vi "LS336_config.vi"(0 "VISA Refnum in":refnum<visa-resource-name>, 1 "Enable Setpoint (F:Off)":bool, 2 "Mode (0:Off)":u16(ring) items=["Off", "Closed Loop PID", "Zone", "Open Loop"], 3 "Rate (D) (0.0 %)":dbl format="%.1f", 4 "Input (0:None)":u16(ring) items=["None", "A", "B", "C", "D"], 5 "Heater Resistance (1:25 Ohms)":u16(ring)=1 items=["25 Ohms"=1, "50 Ohms"=2], 6 "Max Current (0:User Specified)":u16(ring) items=["User Specified", "0.707 A", "1.0 A", "1.141 A", "2.0 A"], 8 "Output's Control Loop (1:1)":u16(ring)=1 items=["1"=1, "2"=2], 9 "Gain (P) (50.0)":dbl=50.0 format="%.1f", 10 "Power Up Enable (F: Off)":bool, 11 "Heater Out Display (1:Current)":u16(ring)=1 items=["Current"=1, "Power"=2], 12 "Manual Output (0.00 %)":dbl format="%.2f", 13 "Max User Current (2.000)":dbl=2.0 format="%.3f", 14 "Range (0:Off)":u16(ring) items=["Off", "Low (On)", "Medium", "High"], 15 "Reset (I) (20.0)":dbl=20.0 format="%.1f", 16 "Setpoint (0.00000)":dbl format="%.5f") -> ()   [LabVIEW 2017]
uses:
  <instrlib>/Lake Shore 336/Lake Shore 336.lvlib
panel:
  in  "Setpoint Ramping \nEnable (F: Off)":bool
  in  "Ramp Rate (0.0)":dbl format="%.1f"
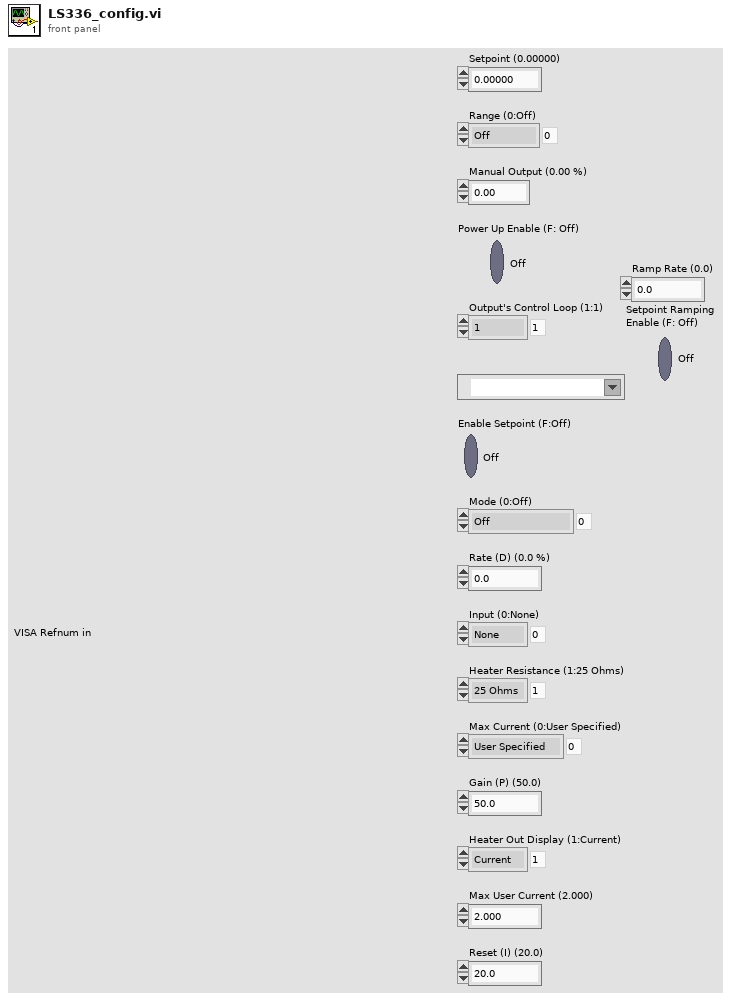
[diagram p1: front panel]
types:
  T1 = cluster{"Baud Rate":u32, "Parity":u16, "Data Bits":u16, "Stop Bits":u16, "Flow Control":u16}
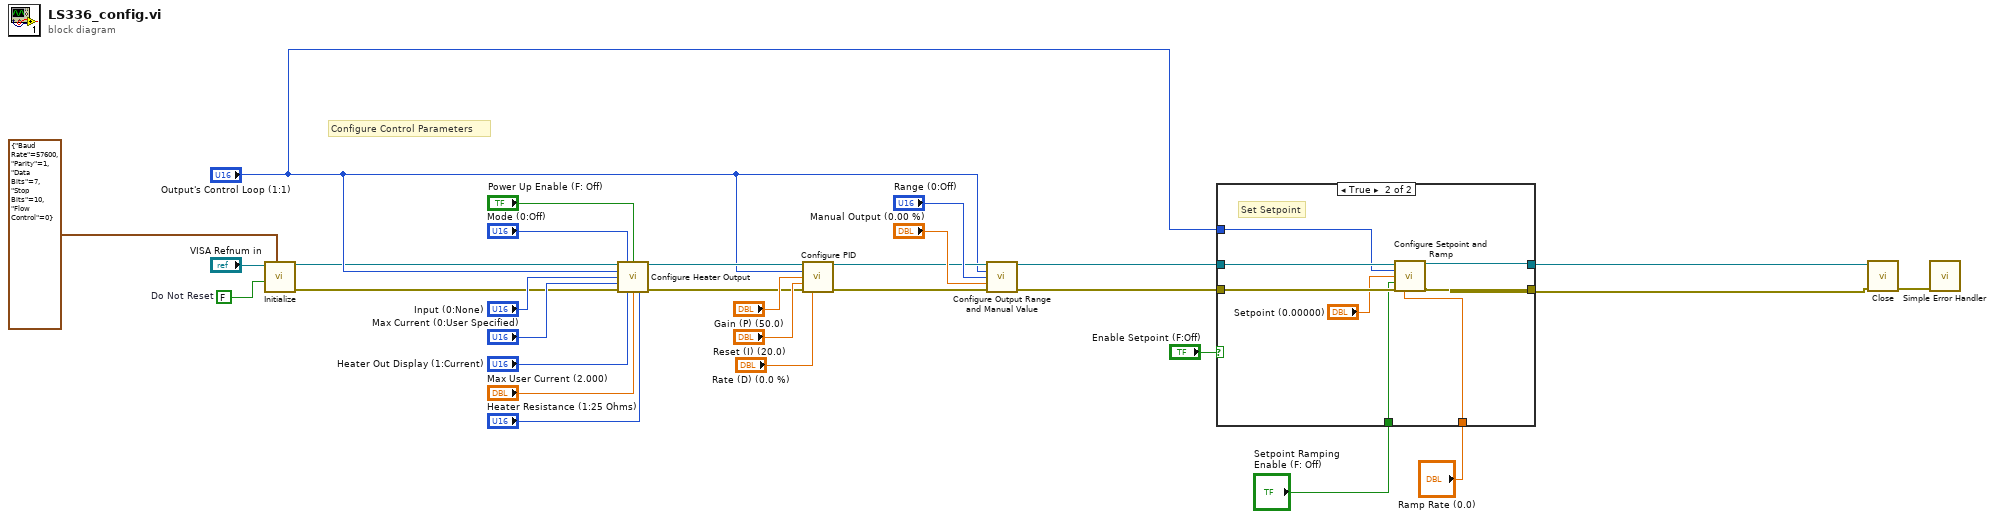
[diagram p0: block diagram]
diagram:
  w10 = FALSE  # Do Not Reset
  # "Configure Control Parameters"
  n1 = call <instrlib>:"Initialize.vi"("Serial Configuration"=T1 {"Baud Rate"=57600, "Parity"=1, "Data Bits"=7, "Stop Bits"=10, "Flow Control"=0}, "Reset (True)"=w10, "VISA resource name"="VISA Refnum in") -> ("error out"=w4:errorcluster, "VISA resource name out"=w3:refnum<visa-resource-name>)  [unwired: 7 in]
  n2 = call <instrlib>:"Configure Heater Output.vi"("VISA resource name"=w3, "Mode (0:Off)"="Mode (0:Off)", "Power Up Enable (F: Off)"="Power Up Enable (F: Off)", "Heater Output (1:1)"="Output's Control Loop (1:1)", "Input (0:None)"="Input (0:None)", "Max Current (0:User Specified)"="Max Current (0:User Specified)", "error in (no error)"=w4, "Heater Out Display (1:Current)"="Heater Out Display (1:Current)", "Max User Current (2.000)"="Max User Current (2.000)", "Heater Resistance (1:25 Ohms)"="Heater Resistance (1:25 Ohms)") -> ("VISA resource name out"=w14:refnum<visa-resource-name>, "error out"=w13:errorcluster)  [unwired: 4 in]
  n3 = call <instrlib>:"Configure PID.vi"("VISA resource name"=w14, "Output's Control Loop (1:1)"="Output's Control Loop (1:1)", "Gain (P) (50.0)"="Gain (P) (50.0)", "Reset (I) (20.0)"="Reset (I) (20.0)", "error in (no error)"=w13, "Rate (D) (0.0 %)"="Rate (D) (0.0 %)") -> ("VISA resource name out"=w15:refnum<visa-resource-name>, "error out"=w16:errorcluster)  [unwired: 8 in]
  n4 = call <instrlib>:"Configure Output Range and Manual Value.vi"("VISA resource name"=w15, "Output (1:1)"="Output's Control Loop (1:1)", "Range (0:Off)"="Range (0:Off)", "Manual Output (0.00 %)"="Manual Output (0.00 %)", "error in (no error)"=w16) -> ("VISA resource name out"=w8:refnum<visa-resource-name>, "error out"=w9:errorcluster)  [unwired: 9 in]
  n5 = case shown="True" "Enable Setpoint (F:Off)" {
    tunnel: "Output's Control Loop (1:1)" -> [_ w38]
    tunnel: w8 -> [w32 w39]
    tunnel: w9 -> [w31 w40]
    tunnel: [w31 w35] -> w30
    tunnel: [w32 w36] -> w29
    tunnel: "Setpoint Ramping \nEnable (F: Off)" -> [_ w34]
    tunnel: "Ramp Rate (0.0)" -> [_ w33]
    frame False {
      # "Do Not Set Setpoint"
    }
    frame True {
      # "Set Setpoint"
      n6 = call <instrlib>:"Configure Setpoint and Ramp.vi"("VISA resource name"=w39, "Output's Control Loop (1:1)"=w38, "Setpoint (0.00000)"="Setpoint (0.00000)", "Setpoint Ramping \nEnable (F: Off)"=w34, "error in (no error)"=w40, "Ramp Rate (0.0)"=w33) -> ("VISA resource name out"=w36:refnum<visa-resource-name>, "error out"=w35:errorcluster)  [unwired: 8 in]
    }
  }
  n7 = call <instrlib>:"Close.vi"("error in (no error)"=w30, "VISA resource name"=w29) -> ("error out"=w7:errorcluster)  [unwired: 9 in]
  n8 = call <vilib>:"Simple Error Handler.vi"("error in (no error)"=w7) -> ()  [unwired: 4 in, 5 out]
